vi "GUI_Bella_BTLsmall.vi"() -> ()   [LabVIEW 2020]
uses:
  Device Drivers/LEPS Interface/Filter_typdef.ctl
  Shared/GUI_Template/GUI_master/tcp_new_data_event.ctl
  Shared/GUI_Template/GUI_master/tcp new data cluster.ctl
  GUI_TestStand/Fire button.ctl
  Device Drivers/DG645/subVIs/TriggerSource_TypDef.ctl
  General GUIs/shared/Image GUI options.ctl
  Controls_pico8752.ctl
panel:
  out "error out":errorcluster
  in  "StepSize.device 1::11":dbl=200.0 caption="Size x" min=0.0 max=100.0
  in  "StepSize.device 2::11":dbl=200.0 caption="Size y" min=0.0 max=100.0
  in  "GUIdevice 11":string="LB-Pico-Booster"
  in  "relativeMove.device 1pos::11":bool
  in  "relativeMove.device 1neg::11":bool
  in  "relativeMove.device 2pos::11":bool
  in  "relativeMove.device 2pos::11":T1
  in  "LPModeSize":cluster{"xhair size":dbl, "xhair size 2":dbl}={"xhair size"=25.0, "xhair size 2"=25.0} {"xhair size 2" min=0.0 max=0.0; "xhair size" min=0.0 max=0.0}
  in  "M5size":cluster{"xhair size":dbl, "xhair size 2":dbl}={"xhair size"=200.0, "xhair size 2"=200.0} {"xhair size 2" min=0.0 max=0.0; "xhair size" min=0.0 max=0.0}
  in  "M4size":cluster{"xhair size":dbl, "xhair size 2":dbl}={"xhair size"=70.0, "xhair size 2"=50.0} {"xhair size 2" min=0.0 max=0.0; "xhair size" min=0.0 max=0.0}
  in  "M2size":cluster{"xhair size":dbl, "xhair size 2":dbl}={"xhair size"=85.0, "xhair size 2"=60.0} {"xhair size 2" min=0.0 max=0.0; "xhair size" min=0.0 max=0.0}
  in  "M1size":cluster{"xhair size":dbl, "xhair size 2":dbl}={"xhair size"=60.0, "xhair size 2"=35.0} {"xhair size 2" min=0.0 max=0.0; "xhair size" min=0.0 max=0.0}
  in  "Stepsize":dbl=0.001 caption="Step Size" min=0.0 max=1.0 format="%.3f"
  in  "Image options 5":T2={"normalize image"=TRUE, "resize and center"=TRUE}
  in  "Image options 4":T2={"normalize image"=TRUE, "resize and center"=TRUE}
  in  "Image options 3":T2={"normalize image"=TRUE, "resize and center"=TRUE}
  in  "Image options 2":T2={"normalize image"=TRUE, "resize and center"=TRUE}
  in  "Image options":T2={"normalize image"=TRUE, "resize and center"=TRUE}
  in  "Trigger.Source::10":T3=enum."External rising edges" caption="SRS Trigger Mode"
  in  "roi::4":bool caption="Blank Button"
  in  "relativeMove.Axis 2neg::6":bool
  in  "relativeMove.Axis 2pos::6":bool
  in  "relativeMove.Axis 3pos::6":bool
  in  "relativeMove.Axis 3neg::6":bool
  in  "trigger::4":bool=TRUE caption="Blank Button"
  in  "exposure::4":dbl=0.0001 caption="Exposure" min=3.8e-05 max=1.0 format="%_4p"
  out "fire::10":string="fire" caption="fire"
  in  "GUIdevice 10":string="BellaSRS"
  in  "Fire Button":T4
  in  "roi::5":bool caption="Blank Button"
  in  "relativeMove.Axis 1neg::8":bool
  in  "relativeMove.Axis 1pos::8":bool
  in  "relativeMove.Axis 2pos::8":bool
  in  "relativeMove.Axis 2neg::8":bool
  in  "trigger::5":bool=TRUE caption="Blank Button"
  in  "exposure::5":dbl=0.4 caption="Exposure" min=3.8e-05 max=1.0 format="%_4p"
  in  "filter.var 2::9":T5=enum."Open(6)" caption="Filter Wheel"
  in  "GUIdevice 5":string="M2Cam"
  out "M2Cam":T6(plugin-control) caption="M1 Cam"
  in  "Target.X::5":dbl=380.0 caption="X" min=0.0 max=2000.0
  in  "Target.Y::5":dbl=360.0 caption="Y" min=0.0 max=2000.0
  in  "GUIdevice 4":string="Bella_LP_Mode"
  out "LPMode":T6(plugin-control) caption="M1 Cam"
  in  "Target.X::4":dbl=700.0 caption="X" min=0.0 max=2000.0
  in  "Target.Y::4":dbl=499.0 caption="Y" min=0.0 max=2000.0
  in  "roi::3":bool caption="Blank Button"
  in  "relativeMove.Axis 1neg::7":bool
  in  "relativeMove.Axis 1pos::7":bool
  in  "relativeMove.Axis 2pos::7":bool
  in  "relativeMove.Axis 2neg::7":bool
  in  "trigger::3":bool=TRUE caption="Blank Button"
  in  "exposure::3":dbl=0.2 caption="Exposure" min=3.8e-05 max=1.0 format="%_4p"
  in  "filter.var 4::9":T5=enum."Open(6)" caption="Filter Wheel"
  in  "GUIdevice 3":string="M4Cam"
  out "M4Cam":T6(plugin-control) caption="M1 Cam"
  in  "Target.X::3":dbl=446.0 caption="X" min=0.0 max=2000.0
  in  "Target.Y::3":dbl=438.0 caption="Y" min=0.0 max=2000.0
  in  "roi::1":bool caption="Blank Button"
  in  "Target.X::1":dbl=582.0 caption="X" min=0.0 max=2000.0
  in  "Target.Y::1":dbl=424.0 caption="Y" min=0.0 max=2000.0
  in  "centroidx::1":dbl caption="X" min=0.0 max=0.0
  in  "centroidy::1":dbl caption="Y" min=0.0 max=0.0
  in  "trigger::1":bool=TRUE caption="Blank Button"
  in  "exposure::1":dbl=0.4 caption="Exposure" min=3.8e-05 max=1.0 format="%_4p"
  in  "filter.var 1::9":T5=enum."Open(6)" caption="Filter Wheel"
  in  "GUIdevice 1":string="M1Cam"
  out "M1Cam":T6(plugin-control) caption="M1 Cam"
  in  "roi::2":bool caption="Blank Button"
  in  "relativeMove.Axis 1pos::6":bool
  in  "relativeMove.Axis 1neg::6":bool
  in  "relativeMove.Axis 3pos::7":bool
  in  "relativeMove.Axis 3neg::7":bool
  in  "trigger::2":bool=TRUE caption="Blank Button"
  in  "exposure::2":dbl=0.8 caption="Exposure" min=3.8e-05 max=1.0 format="%_4p"
  in  "GUIdevice 2":string="M5Cam"
  in  "filter.var 5::9":T5=enum."Open(6)" caption="Filter Wheel"
  out "M5Cam":T6(plugin-control) caption="M1 Cam"
  out "stepsize::6":dbl=0.01 caption="Step Size" min=0.0 max=1.0 format="%.3f"
  out "stepsize::7":dbl=0.01 caption="Step Size" min=0.0 max=1.0 format="%.3f"
  out "stepsize::8":dbl=0.01 caption="Step Size" min=0.0 max=1.0 format="%.3f"
  in  "Target.X::2":dbl=804.0 caption="X" min=0.0 max=2000.0
  in  "Target.Y::2":dbl=608.0 caption="Y" min=0.0 max=2000.0
  in  "GUIdevice 9":string="71146 LEPS Interface"
  out "tcp data event":T7
  in  "GUIdevice 8":string="BELLA_ESP_M1"
  in  "GUIdevice 7":string="BellaESP"
  in  "GUIdevice 6":string="BELLA_ESP_2"
  in  "stop":bool
  out "error IO 2":errorcluster
  # "Target"
  # "Target"
  # "Target"
  # "Centroid"
  # "M5 X-Axis, LP Mode CAMS"
  # "M5 Y-Axis, M4 CAMS"
  # "M2 CAM"
  # "M5 and LP Mode CAMS"
  # "M4 and M5 CAMS"
  # "M2 CAM"
  # "Target"
  # "Target"
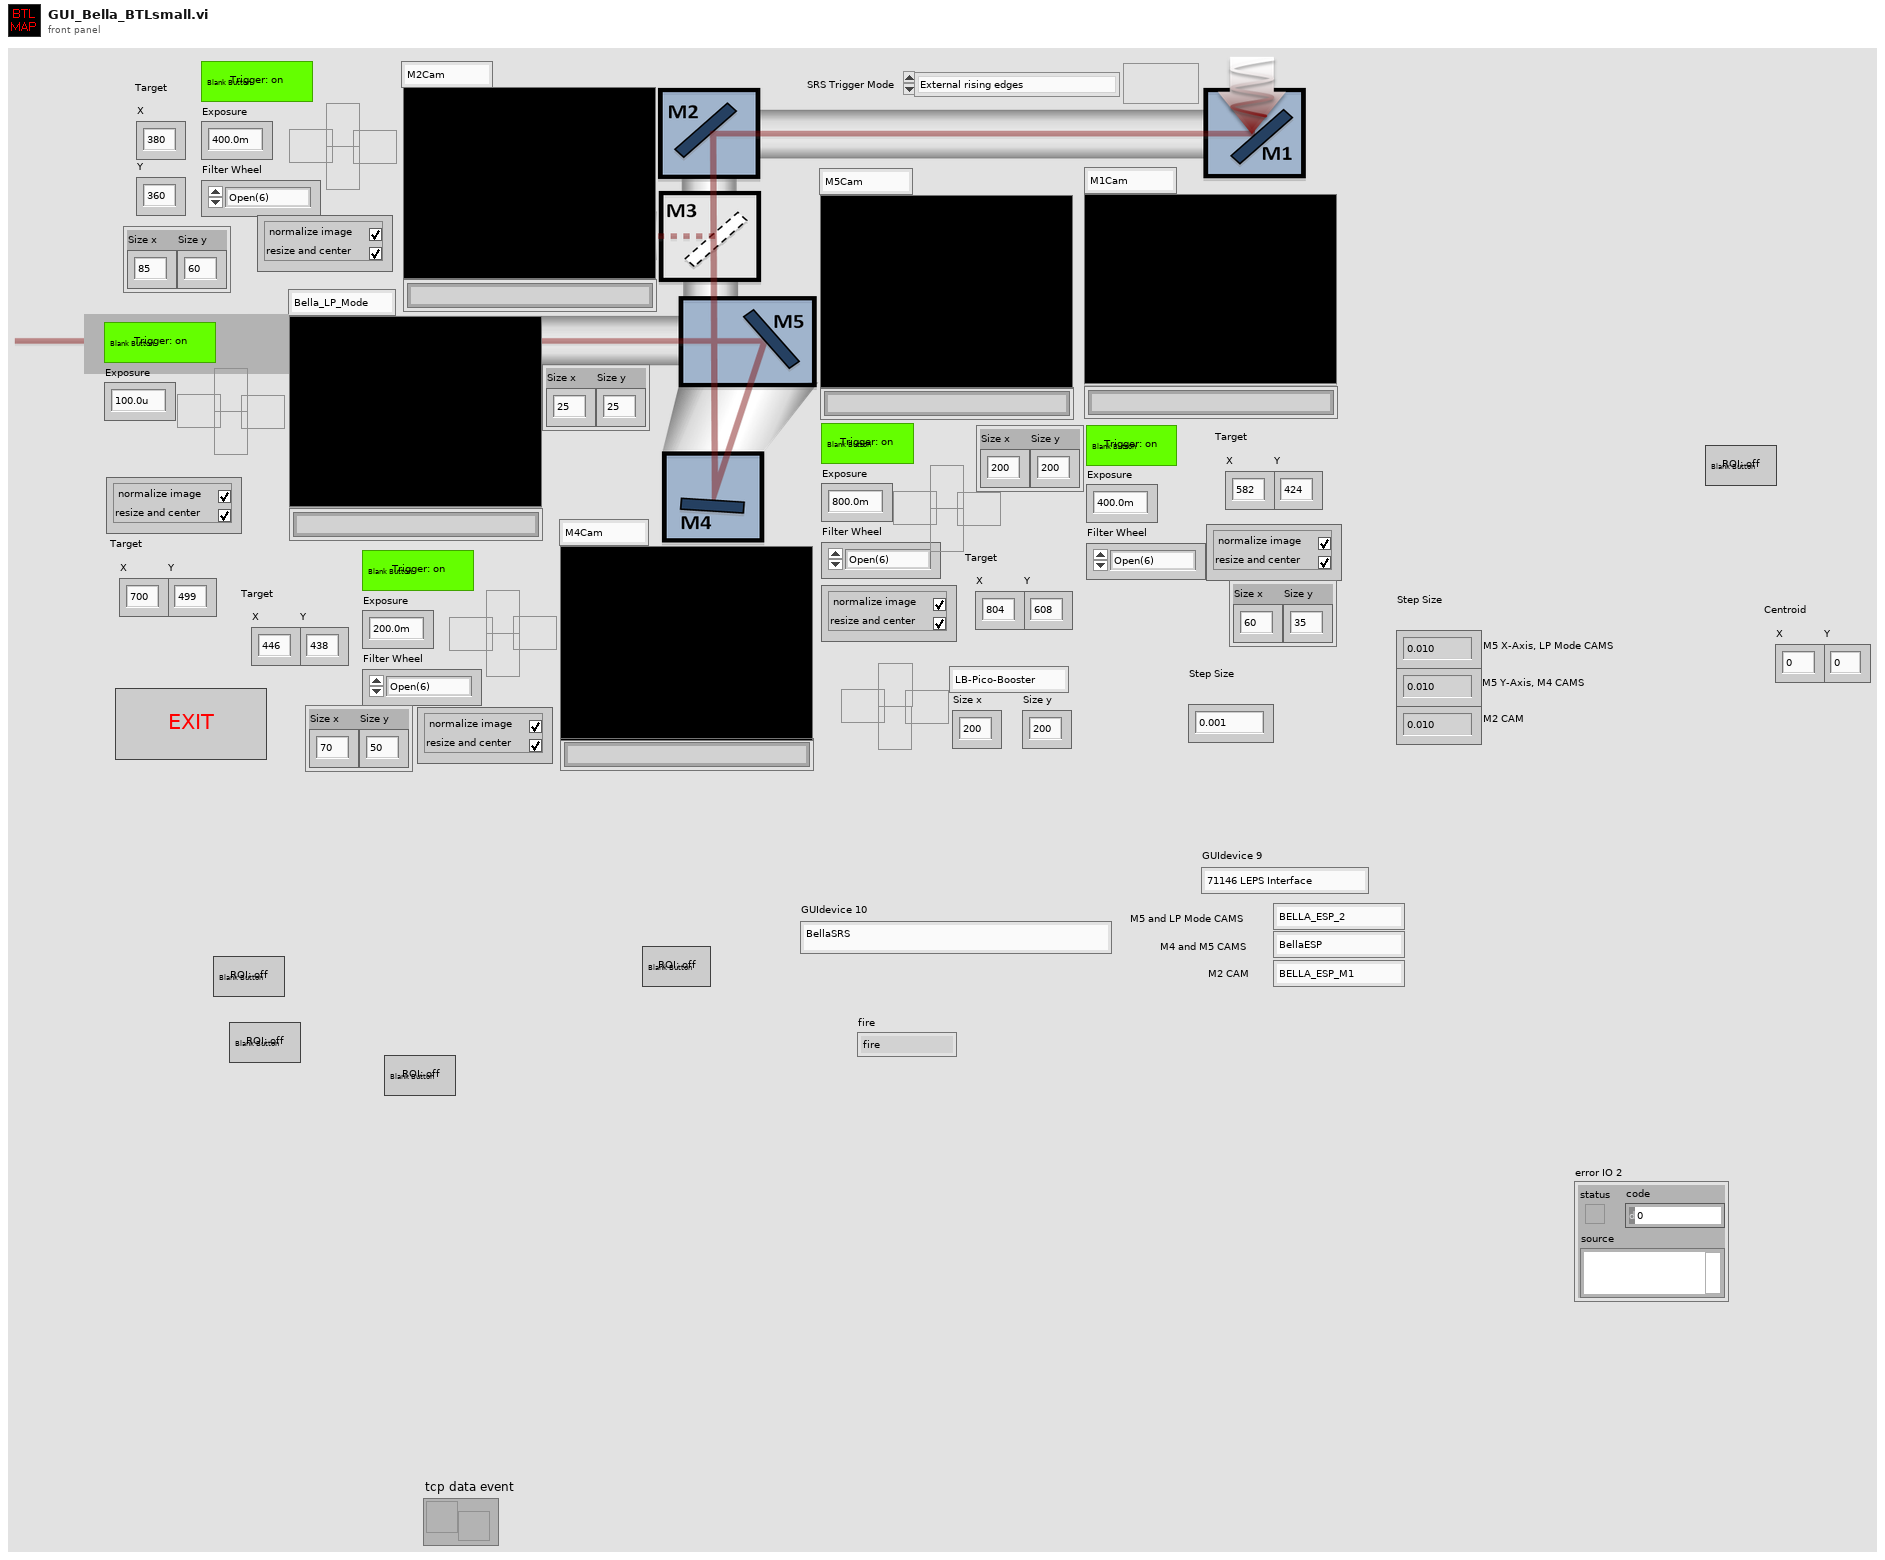
[diagram p1: front panel]
types:
  T1 = typedef "Controls_pico8752.ctl" = bool
  T2 = typedef "Image GUI options.ctl" = cluster{"normalize image":bool, "resize and center":bool}
  T3 = typedef "TriggerSource_TypDef.ctl" = enum16{"Internal", "External rising edges", "External falling edges", "Single shot external rising edges", "Single shot external falling edges", "Single shot", "Line"}
  T4 = typedef "Fire button.ctl" = bool
  T5 = typedef "Filter_typdef.ctl" = enum16{"Moving/Unknown", "OD1", "OD2", "OD3", "OD4", "OD5", "Open(6)"}
  T6 = typedef "IMAQ Image.ctl" = refnum<image>
  T7 = typedef "tcp_new_data_event.ctl" = refnum<user-event>
  T8 = typedef "tcp new data cluster.ctl" = cluster{"EventEnum":enum16{"new data", "connection status update"}, "Device name":string}
  T9 = typedef "Image Type" = u32
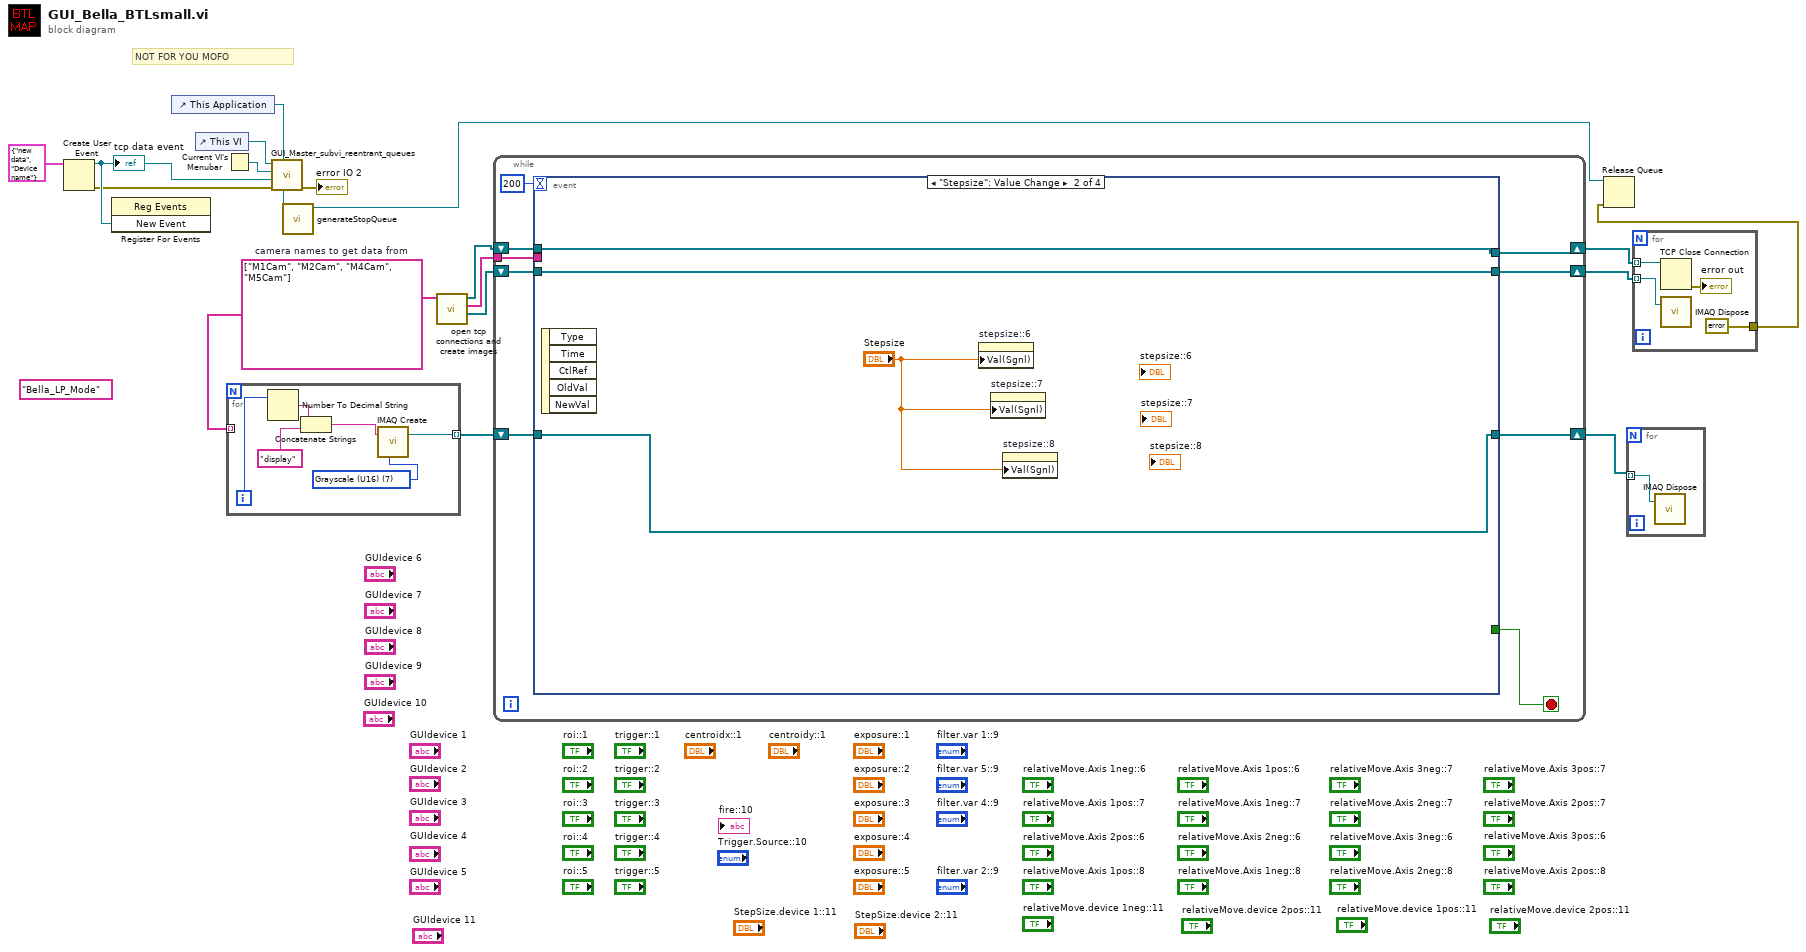
[diagram p0: block diagram]
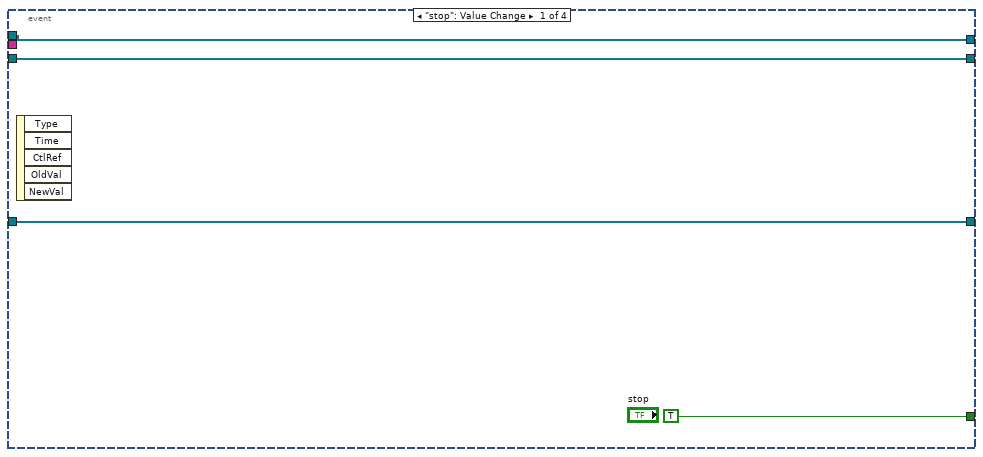
[diagram p2: hidden frame]
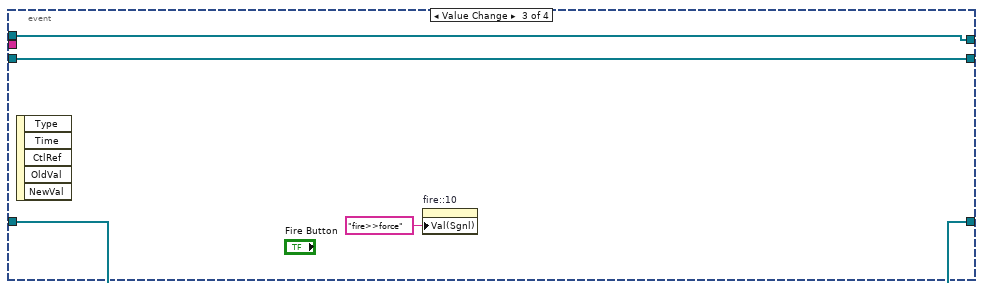
[diagram p3: hidden frame]
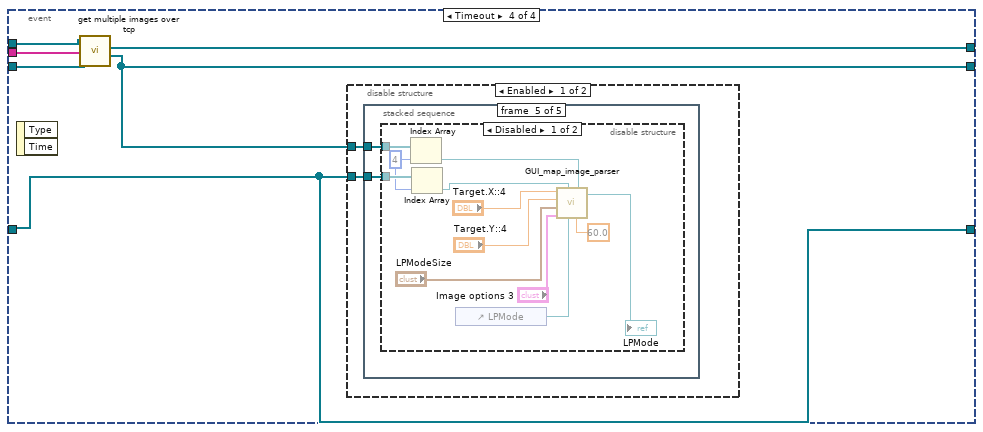
[diagram p4: hidden frame]
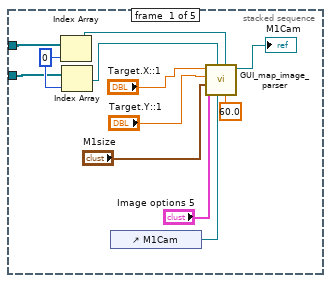
[diagram p5: hidden frame]
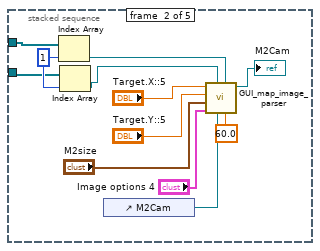
[diagram p6: hidden frame]
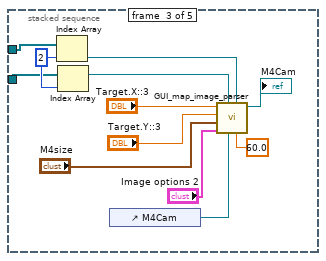
[diagram p7: hidden frame]
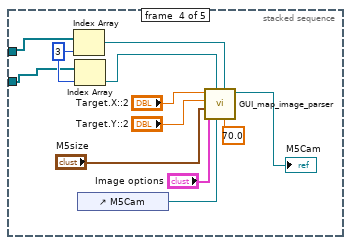
[diagram p8: hidden frame]
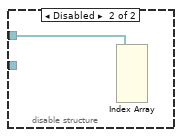
[diagram p10: hidden frame]
diagram:
  (unwired) "Bella_LP_Mode"
  w5 = string[] ["M1Cam", "M2Cam", "M4Cam", "M5Cam"]  # camera names to get data from
  # "NOT FOR YOU MOFO"
  n1 = Create User Event(user event datatype=T8 {"EventEnum"=enum."new data", "Device name"="Device name"} ("New Event")) -> (user event=w16:refnum<user-event>, error out=w15:errorcluster)  [unwired: 1 in]
  "tcp data event" <- w16
  n2 = register-events(w16) -> ()  [unwired: 2 in, 2 out]
  n3 = control-ref of="This Application"() -> (w17:refnum<vi>)
  n4 = control-ref of="This VI"() -> (w12:refnum<vi>)
  n5 = Current VI's Menubar() -> (w13:refnum<k9>)
  n6 = for {
    tunnel: w5 -> [_] mode=indexing
    tunnel: [w21] -> w4 mode=indexing
    i -> [w19]
    w23 = T9 7 items=["Grayscale (U8)", "Grayscale (I16)", "Grayscale (SGL)", "Complex (CSG)", "RGB (U32)", "HSL (U32)", "RGB (U64)", "Grayscale (U16)"] ("Image Type")
    n7 = Number To Decimal String(number=w19) -> (decimal integer string=w18:string)  [unwired: 1 in]
    n8 = Concatenate Strings(w18, "display" ("string")) -> (w22:string)
    n9 = call "IMAQ Create"("Image Name"=w22, "Image Type"=w23) -> ("New Image"=w21:T6)  [unwired: 3 in, 1 out]
  }
  n10 = call "generateStopQueue.vi"() -> ("STOP Queue out"=w2:refnum<queue>)  [unwired: 10 in, 1 out]
  n11 = call "GUI_Master_subvi_reentrant_queues.vi"("STOP Queue in"=w2, "This Application"=w17, "error in (no error)"=w15, "tcp data event"=w16, "Caller menu reference"=w13, "Caller VI ref"=w12) -> ("error out"=→"error IO 2":errorcluster)  [unwired: 5 in]
  n12 = call "open tcp connections and create images.vi"("devices to get data from"=w5) -> ("images"=w9:T6[], "subscribe messages\nfor process vis"=w6:string[], "tcp connections"=w10:refnum<k5>[])  [unwired: 8 in]
  n13 = while {
    shift-right: [w28] -> w8
    shift-left: w10 -> [w30]
    shift-right: [w27] -> w7
    shift-left: w9 -> [w29]
    tunnel: w6 -> [w26]
    shift-right: [w24] -> w3
    shift-left: w4 -> [w25]
    stop <- w32 stop-if-true
    n14 = event shown="[1] \"Stepsize\": Value Change" {
      selector: _ -> [_ _ _ _]
      dyn-events: _ -> [_ _ _ _]
      timeout: 200 -> [_ _ _ _]
      tunnel: [TRUE ("stop") _ _ _] -> w32
      tunnel: w30 -> [w35 w39 w43 w50]
      tunnel: w29 -> [w34 w38 w42 w49]
      tunnel: [w35 w39 w43 w48] -> w28
      tunnel: [w34 w38 w42 w46] -> w27
      tunnel: w26 -> [_ _ _ w47]
      tunnel: w25 -> [w33 w37 w41 w45]
      tunnel: [w33 w37 w41 w45] -> w24
      event "stop": Value Change {
        n15 = event-data() -> ()  [unwired: 1 in, 5 out]
      }
      event "Stepsize": Value Change {
        n16 = event-data() -> ()  [unwired: 1 in, 5 out]
        n17 = property on="stepsize::6" class="DigNum (strict)"("Val(Sgnl)"="Stepsize") -> ()  [unwired: 2 in, 2 out]
        n18 = property on="stepsize::7" class="DigNum (strict)"("Val(Sgnl)"="Stepsize") -> ()  [unwired: 2 in, 2 out]
        n19 = property on="stepsize::8" class="DigNum (strict)"("Val(Sgnl)"="Stepsize") -> ()  [unwired: 2 in, 2 out]
      }
      event Value Change {
        n20 = event-data() -> ()  [unwired: 1 in, 5 out]
        n21 = property on="fire::10" class="Str"("Val(Sgnl)"="fire>>force" ("Value (Signaling)")) -> ()  [unwired: 2 in, 2 out]
      }
      event Timeout {
        n22 = event-data() -> ()  [unwired: 1 in, 2 out]
        n23 = call "get multiple images over tcp.vi"("images In"=w49, "subscribeMessages"=w47, "TCP_Refs In"=w50) -> ("Images out"=w46:T6[], "TCP_Refs_out"=w48:refnum<k5>[])  [unwired: 4 in, 3 out]
        n24 = disable-structure shown="Enabled" {
          disable-tunnel: w46 -> [w52 w120]
          disable-tunnel: w45 -> [w51 _]
          frame Enabled {
            n25 = stacked-sequence {
              tunnel: w52 -> [w58 w70 w82 w94 w102]
              tunnel: w51 -> [w57 w69 w81 w93 w101]
              frame #0 {
                w59 = 0 ("index")
                n26 = Index Array(array=w58, index=w59) -> (element=w56:T6)
                n27 = Index Array(array=w57, index=w59) -> (element=w55:T6)
                n28 = control-ref of="M1Cam"() -> (w62:refnum<vi>)
                n29 = call "GUI_map_image_parser.vi"("zoom#"=60.0, "Image Src"=w56, "Ctl Refnum"=w62, "Image Dst"=w55, "Image options"="Image options 5", "size"="M1size", "target y"="Target.Y::1", "target x"="Target.X::1") -> ("Img out"=→"M1Cam":T6)  [unwired: 2 in, 1 out]
              }
              frame #1 {
                w71 = 1 ("index")
                n30 = Index Array(array=w70, index=w71) -> (element=w68:T6)
                n31 = Index Array(array=w69, index=w71) -> (element=w67:T6)
                n32 = control-ref of="M2Cam"() -> (w74:refnum<vi>)
                n33 = call "GUI_map_image_parser.vi"("zoom#"=60.0, "Image Src"=w68, "Ctl Refnum"=w74, "Image Dst"=w67, "Image options"="Image options 4", "size"="M2size", "target y"="Target.Y::5", "target x"="Target.X::5") -> ("Img out"=→"M2Cam":T6)  [unwired: 2 in, 1 out]
              }
              frame #2 {
                w83 = 2 ("index")
                n34 = Index Array(array=w82, index=w83) -> (element=w80:T6)
                n35 = Index Array(array=w81, index=w83) -> (element=w79:T6)
                n36 = control-ref of="M4Cam"() -> (w85:refnum<vi>)
                n37 = call "GUI_map_image_parser.vi"("zoom#"=60.0, "Image Src"=w80, "Ctl Refnum"=w85, "Image Dst"=w79, "Image options"="Image options 2", "size"="M4size", "target y"="Target.Y::3", "target x"="Target.X::3") -> ("Img out"=→"M4Cam":T6)  [unwired: 2 in, 1 out]
              }
              frame #3 {
                w95 = 3 ("index")
                n38 = Index Array(array=w94, index=w95) -> (element=w92:T6)
                n39 = Index Array(array=w93, index=w95) -> (element=w91:T6)
                n40 = control-ref of="M5Cam"() -> (w99:refnum<vi>)
                n41 = call "GUI_map_image_parser.vi"("zoom#"=70.0, "Image Src"=w92, "Ctl Refnum"=w99, "Image Dst"=w91, "Image options"="Image options", "size"="M5size", "target y"="Target.Y::2", "target x"="Target.X::2") -> ("Img out"=→"M5Cam":T6)  [unwired: 2 in, 1 out]
              }
              frame #4 {
                n42 = disable-structure shown="Disabled" {
                  disable-tunnel: w102 -> [w109 _]
                  disable-tunnel: w101 -> [w107 _]
                  frame Disabled {
                    w105 = 4 ("index")
                    n43 = Index Array(array=w109, index=w105) -> (element=w108:T6)
                    n44 = Index Array(array=w107, index=w105) -> (element=w106:T6)
                    n45 = control-ref of="LPMode"() -> (w112:refnum<vi>)
                    n46 = call "GUI_map_image_parser.vi"("zoom#"=60.0, "Image Src"=w108, "Ctl Refnum"=w112, "Image Dst"=w106, "Image options"="Image options 3", "size"="LPModeSize", "target y"="Target.Y::4", "target x"="Target.X::4") -> ("Img out"=→"LPMode":T6)  [unwired: 2 in, 1 out]
                  }
                  frame Enabled {
                  }
                }
              }
            }
          }
          frame Disabled {
            n47 = Index Array(array=w120) -> (element #1=w119:T6, element #2=w118:T6, element #3=w117:T6, element #4=w116:T6, element #5=w115:T6)  [unwired: 5 in]
          }
        }
      }
    }
  }
  n48 = for {
    tunnel: w3 -> [w121] mode=indexing
    n49 = call "IMAQ Dispose"("Image"=w121) -> ()  [unwired: 5 in, 1 out]
  }
  n50 = for {
    tunnel: w8 -> [w125] mode=indexing
    tunnel: w7 -> [w124] mode=indexing
    tunnel: [errorcluster {"status"=FALSE, "code"=0, "source"=""} ("error in (no error)")] -> w1
    n51 = TCP Close Connection(connection ID=w125) -> (error out=→"error out":errorcluster)  [unwired: 2 in, 1 out]
    n52 = call "IMAQ Dispose"("Image"=w124) -> ()  [unwired: 5 in, 1 out]
  }
  n53 = Release Queue(queue=w2, error in (no error)=w1) -> ()  [unwired: 1 in, 3 out]
